vi "Example2.vi"() -> ()   [LabVIEW 2017]
uses:
  FP Publisher/Front Panel Publisher.lvlib
  FP Publisher/Common/Enum - Config Option.ctl
  FP Publisher/Web Front Panel_class/Controls/High Level Config Settings.ctl
  FP Publisher/Web Front Panel_class/Web Front Panel.lvclass
  FP Publisher/Web Front Panel_class/Controls/Cluster - Default Control Behavior.ctl
  <vilib>/Platform/browser.llb/Open URL in Default Browser (path).vi
panel:
  in  "Stop":bool
  out "XY Graph":cluster{i32[], dbl[]}(graph)
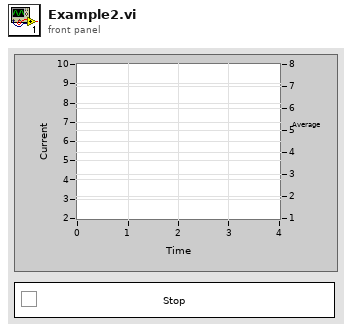
[diagram p1: front panel]
types:
  T1 = typedef "Front Panel Publisher.lvlib/Web Front Panel.lvclass/Cluster - Default Control Behavior.ctl" = cluster{"Value Controls":string[], "Value and Position Controls":string[], "Image Controls":string[], "Image and Position Controls":string[]}
  T2 = typedef "Front Panel Publisher.lvlib/Web Front Panel.lvclass/High Level Config Settings.ctl" = cluster{"Default Refresh Rate (ms)":i32, "Show Border":bool, "Periodic Decoration Data":bool, "Synchronous Requests":bool, "Reduce Sent Data":bool, "Recommended Control Settings":bool}
  T3 = typedef "Front Panel Publisher.lvlib/Enum - Config Option.ctl" = enum16{"Show Config Dialog", "Don't Show Config Dialog", "Load Config File then Show Dialog", "Load Config File No Dialog"}
  T4 = typedef "LVPointTypeDef.ctl" = cluster{"Horizontal":i16, "Vertical":i16}
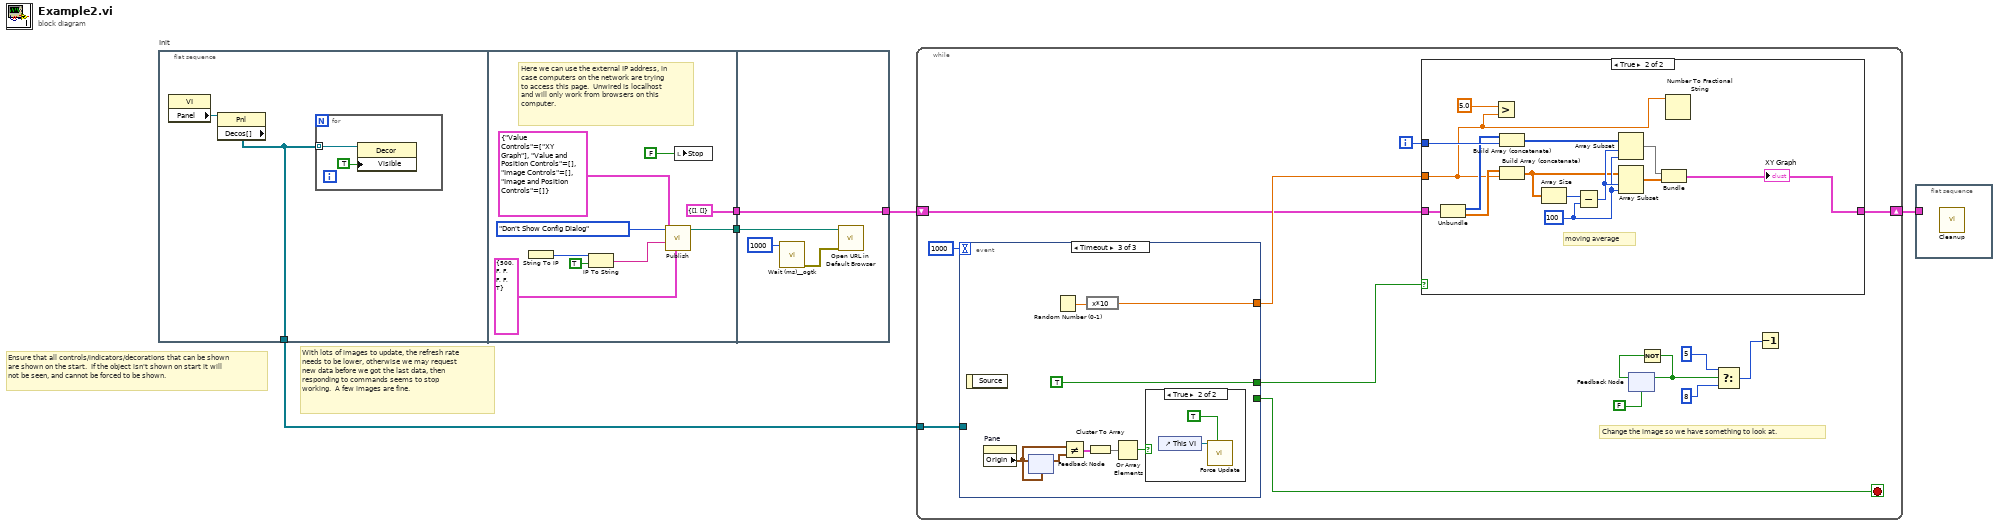
[diagram p0: block diagram]
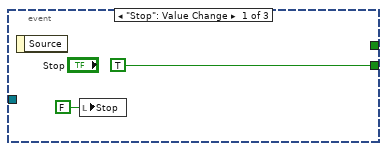
[diagram p3: hidden frame]
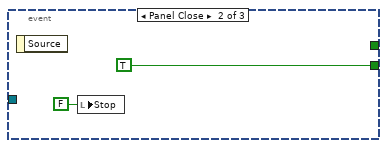
[diagram p4: hidden frame]
diagram:
  # "Ensure that all controls/indicators/decorations that can be shown are shown on the start.  If the object isn't shown on start it will not be seen, and cannot be forced to be shown."
  # "With lots of images to update, the refresh rate needs to be lower, otherwise we may request new data before we got the last data, then responding to commands seems to stop working.  A few images are fine."
  n1 = flat-sequence "Init" {
    tunnel: [w6] -> w1
    tunnel: [cluster{i32[], dbl[]} {[], []} ("XY Graph")] -> w5
    tunnel: [w14] -> w4
    tunnel: [w22] -> w3
    tunnel: w5 -> [w22]
    tunnel: w4 -> [w21]
    frame #0 {
      n2 = property class="VI"() -> ("Panel"=w7:refnum<vi>)  [unwired: 2 in, 2 out]
      n3 = property class="Pnl"(reference=w7) -> ("Decos[]"=w6:refnum<vi>[])  [unwired: 1 in, 2 out]
      n4 = for {
        tunnel: w6 -> [w8] mode=indexing
        n5 = property class="Decor"(reference=w8, "Visible"=TRUE) -> ()  [unwired: 1 in, 2 out]
      }
    }
    frame #1 {
      # "Here we can use the external IP address, in case computers on the network are trying to access this page.  Unwired is localhost and will only work from browsers on this computer."
      n6 = String To IP() -> (0:w15:u32)  [unwired: 1 in]
      n7 = IP To String(1:TRUE ("dot notation? (F)"), 2:w15) -> (0:w12:string)
      n8 = call "Publish.vi"("High Level Config Settings"=T2 {"Default Refresh Rate (ms)"=500, "Show Border"=FALSE, "Periodic Decoration Data"=FALSE, "Synchronous Requests"=FALSE, "Reduce Sent Data"=FALSE, "Recommended Control Settings"=TRUE}, "Host Connection"=w12, "Default Control Behavior"=T1 {"Value Controls"=["XY Graph"], "Value and Position Controls"=[], "Image Controls"=[], "Image and Position Controls"=[]}, "Config Option"=Enum_-_Config_Option."Don't Show Config Dialog") -> ("Created HTML"=w14:path)  [unwired: 5 in, 2 out]
      n9 = local write "Stop"(FALSE ("Stop")) -> ()
    }
    frame #2 {
      n10 = call <userlib>:"Wait (ms)__ogtk.vi"("milliseconds to wait"=u32 1000) -> ("error out"=w20:errorcluster)  [unwired: 9 in, 1 out]
      n11 = call-poly <vilib>:"Open URL in Default Browser.vi"("error in (no error)"=w20, "path"=w21) -> ()  [unwired: 4 in, 2 out]
    }
  }
  n12 = while {
    shift-right: [w31] -> w2
    shift-left: w3 -> [w30]
    tunnel: w1 -> [w24]
    i -> [w33]
    stop <- w36 stop-if-true
    # "Change the image so we have something to look at."
    n13 = event shown="[2] Timeout" {
      selector: _ -> [_ _ _]
      dyn-events: _ -> [_ _ _]
      timeout: 1000 -> [_ _ _]
      tunnel: [TRUE TRUE _] -> w36
      tunnel: [_ _ w62] -> w32
      tunnel: [_ _ TRUE] -> w34
      tunnel: w24 -> [_ _ _]
      event "Stop": Value Change {
        n14 = event-data() -> ()  [unwired: 1 in, 1 out]
        n15 = local write "Stop"(FALSE ("Stop")) -> ()
      }
      event Panel Close {
        n16 = event-data() -> ()  [unwired: 1 in, 1 out]
        n17 = local write "Stop"(FALSE ("Stop")) -> ()
      }
      event Timeout {
        n18 = event-data() -> ()  [unwired: 1 in, 1 out]
        n19 = property on="Pane" class="Pane"() -> ("Origin"=w59:T4)  [unwired: 2 in, 2 out]
        n20 = feedback-in #1(w59) -> ()
        n21 = feedback #1(w59) -> (w60:T4)
        n22 = Random Number (0-1)() -> (number: 0 to 1=w63:dbl)
        n23 = Not Equal?(x=w59, y=w60) -> (x != y?=w58:cluster{"Horizontal":bool, "Vertical":bool})
        n24 = expression code="x*10"(w63) -> (w62:dbl)
        n25 = Cluster To Array(cluster=w58) -> (array=w57:bool[])
        n26 = Or Array Elements(Boolean array=w57) -> (logical OR=w56:bool)
        n27 = case shown="True" w56 {
          frame False {
          }
          frame True {
            n28 = control-ref of="This VI"() -> (w65:refnum<vi>)
            n29 = call "Force Update.vi"("Update Origin"=TRUE, "VI Refnum"=w65) -> ()  [unwired: 10 in]
          }
        }
      }
    }
    n30 = case shown="True" w34 {
      tunnel: w33 -> [_ w51]
      tunnel: w32 -> [_ w39]
      tunnel: [w37 w38] -> w31
      tunnel: w30 -> [w37 w50]
      frame False {
      }
      frame True {
        w45 = 100 ("length")
        # "moving average"
        n31 = Unbundle(w50) -> (w48:i32[], w44:dbl[])
        n32 = Greater?(x=5.0, y=w39) -> ()  [unwired: 1 out]
        n33 = Build Array (concatenate)(w48, w51) -> (w49:i32[])
        n34 = Build Array (concatenate)(w44, w39) -> (w43:dbl[])
        n35 = Array Size(array=w43) -> (size(s)=w47:i32)
        n36 = Subtract(x=w47, y=w45) -> (x-y=w46:i32)
        n37 = Array Subset(array=w49, index=w46, length=w45) -> (w41:i32[])
        n38 = Array Subset(array=w43, index=w46, length=w45) -> (w40:dbl[])
        n39 = Bundle(w41, w40) -> (w38:cluster{i32[], dbl[]})  [unwired: 1 in]
        "XY Graph" <- w38
        n40 = Number To Fractional String(number=w39) -> ()  [unwired: 3 in, 1 out]
      }
    }
    n41 = feedback #2(FALSE) -> (w28:bool)
    n42 = Not(x=w28) -> (.not. x?=w25:bool)
    n43 = feedback-in #2(w25) -> ()
    n44 = Select(t=u32 5 ("Number of Rows"), s=w25, f=u32 8 ("Number of Rows")) -> (s? t:f=w23:u32)
    n45 = Decrement(x=w23) -> ()  [unwired: 1 out]
  }
  n46 = flat-sequence {
    tunnel: w2 -> [_]
    frame #0 {
      n47 = call "Cleanup.vi"() -> ()  [unwired: 11 in, 1 out]
    }
  }
